vi "Launcher.vi"() -> ()   [LabVIEW 2014, in "HIJ Multiple Cams App Demo.lvlib"]
uses:
  HIJ Multiple Cams App Demo.lvlib
  <vilib>/userdefined/High Color/IMAQdx.ctl
  HIJ Multiple Cams App Demo/HIJ Multiple Cams App Demo.lvclass
  HIJ Multiple Cams App Demo/HIJ Multiple Cams App Demo.lvclass/HIJ Multiple Cams App Demo.ctl
  HIJ Multiple Cams App Demo/Write Start Camera 1.vi
  HIJ Multiple Cams App Demo/Write Start ConfigDir.vi
  HIJ Multiple Cams App Demo/Write Start WorkDir.vi
  HIJ Multiple Cams App Demo/Write Start Camera 2.vi
  <vilib>/ActorFramework/Actor/Actor.lvclass
panel:
  in  "Start Camera 2":T1="dummy"
  in  "Start WorkDir":path=path "C:/Users/user/Desktop/test/WorkDir"
  in  "Start ConfigDir":path=path "C:/Users/user/Desktop/test/ConfigDir"
  in  "Start Camera 1":T1="TestCam"
  out "error out":errorcluster
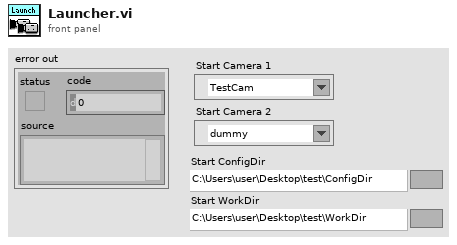
[diagram p1: front panel]
types:
  T1 = typedef "IMAQdx.ctl" = refnum<k21>
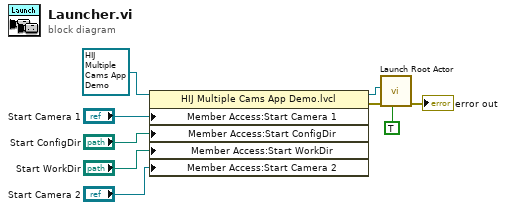
[diagram p0: block diagram]
diagram:
  n1 = property class="HIJ Multiple Cams App Demo.lvcl"(reference=refnum<class "HIJ Multiple Cams App Demo.lvclass"> refnum ("HIJ Multiple Cams App Demo.lvlib:HIJ Multiple Cams App Demo.lvclass"), "Member Access:Start Camera 1"="Start Camera 1", "Member Access:Start ConfigDir"="Start ConfigDir", "Member Access:Start WorkDir"="Start WorkDir", "Member Access:Start Camera 2"="Start Camera 2") -> (reference out=w8:refnum<class "HIJ Multiple Cams App Demo.lvclass">, error out=w7:errorcluster)  [unwired: 1 in]
  n2 = call <vilib>:"Launch Root Actor.vi"("Open Actor Core front panel? (F)"=TRUE, "error in (no error)"=w7, "Actor"=w8) -> ("error out"=→"error out":errorcluster)  [unwired: 7 in, 1 out]
